vi "Analog Write N Chans.vi"(7 "Analog Ref Override":dbl, 8 "Error In":errorcluster, 9 "AO Values":dbl[](array[numeric]), 10 "AO Channel(s)":u8[](array[numeric]), 11 "LINX Resource":T1) -> (0 "Error Out":errorcluster, 3 "LINX Resource":T1)   [LabVIEW 2014, in "LMH-LINX.lvlib"]
doc: "Write value(s) to the specified analog output channel(s)."
uses:
  <vilib>/MakerHub/LINX/LMH-LINX.lvlib
  <vilib>/MakerHub/LINX/Private/Type Defs/LINX Ref.ctl
  <vilib>/MakerHub/LINX/Private/Type Defs/Platform.ctl
  <vilib>/MakerHub/LINX/Private/Type Defs/Interface.ctl
  <vilib>/MakerHub/LINX/Private/Device/Type Defs/LINX Device Config.ctl
  <vilib>/MakerHub/LINX/Private/Device/Type Defs/TCP Config.ctl
  <vilib>/MakerHub/LINX/Private/Device/Type Defs/Channels.ctl
  <vilib>/MakerHub/LINX/Private/Type Defs/Peripheral.ctl
  <vilib>/MakerHub/LINX/Private/Utilties/Generate Error.vi
  <vilib>/myRIO/Common/Instrument Driver Framework/myRIO v1.0/AO/vis/myRIO v1.0 Write AO.vi
  <vilib>/Utility/error.llb/Error Cluster From Error Code.vi
  <vilib>/MakerHub/LINX/Private/myRIO/myRIO.lvlib
  <vilib>/MakerHub/LINX/Private/Device/Device.lvlib
  <vilib>/myRIO/Instrument Drivers/Onboard IO/AO/AO.lvlib
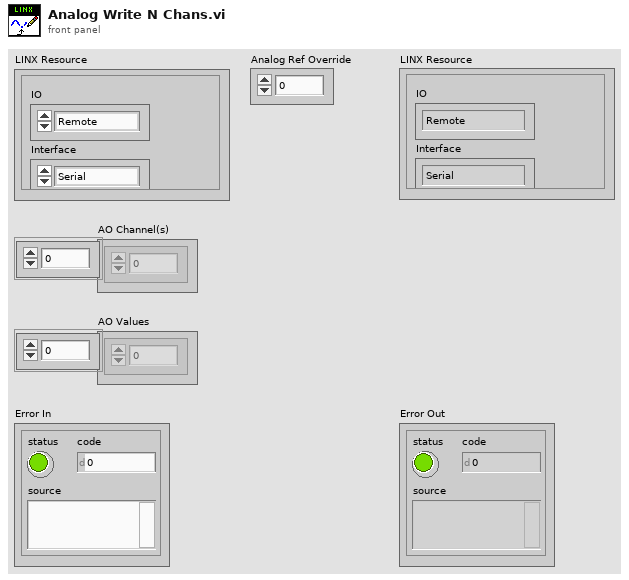
[diagram p1: front panel]
types:
  T1 = typedef "LMH-LINX.lvlib/LINX Ref.ctl" = cluster{"IO":T2, "Interface":T3, "LINX Device Config":T4}
  T2 = typedef "LMH-LINX.lvlib/Platform.ctl" = enum16{"Remote", "Local"}
  T3 = typedef "LMH-LINX.lvlib/Interface.ctl" = enum16{"Serial", "TCP"}
  T4 = typedef "LMH-LINX.lvlib/Device.lvlib/LINX Device Config.ctl" = cluster{"Interface":T3, "COM Port":refnum<visa-resource-name>, "TCP Configuration":T5, "Device Family":u8, "Device ID":u8, "Device Name":string, "TCP Ref":refnum<k5>, "Channels":T6}
  T5 = typedef "LMH-LINX.lvlib/Device.lvlib/TCP Config.ctl" = cluster{"IP Address":string, "Port":u16}
  T6 = typedef "LMH-LINX.lvlib/Channels.ctl" = cluster{"DI":u8[], "DO":u8[], "AI":u8[], "AO":u8[], "PWM":u8[], "QE":u8[], "UART":u8[], "I2C 2":u8[], "SPI":u8[], "CAN":u8[], "Servo":u8[], "AI Ref (V)":dbl, "AI Resolution (Bits)":u8, "AO Ref (V)":dbl, "AO Resolution (Bits)":u8}
  T7 = typedef "LMH-LINX.lvlib/Peripheral.ctl" = enum8{"DI", "DO", "AI", "AO", "PWM", "QE", "UART", "I2C", "SPI", "CAN", "Servo"}
  T8 = typedef "AO.lvlib/AO Reference.ctl" = cluster{"myRIO Reference":T9, "AO Channel List":T13, "AO Scaling Constant List":T15}
  T9 = typedef "myRIO Generic Hardware Reference.ctl" = cluster{"myRIO Model":T10, "myRIO Hardware Reference":T11}
  T10 = typedef "Hardware Version Enum.ctl" = enum16{"Unknown", "myRIO-1900", "myRIO-1950"}
  T11 = typedef "myRIO v1.0 Reference.ctl" = cluster{"Generic FPGA Reference":T12, "Allow multiple opens":bool}
  T12 = typedef "Generic FPGA Reference.ctl" = refnum<k20>
  T13 = typedef "AO Channels List.ctl" = T14[]
  T14 = typedef "AO Channels Enum.ctl" = enum16{"Not Connected", "AudioOut/Left", "AudioOut/Right", "C/AO0", "C/AO1", "A/AO0", "A/AO1", "B/AO0", "B/AO1"}
  T15 = typedef "Analog Scaling Constants List.ctl" = T16[]
  T16 = typedef "Analog Scaling Constants.ctl" = cluster{"LSB Weight (Volts)":dbl, "Offset (Volts)":dbl, "Signed?":bool}
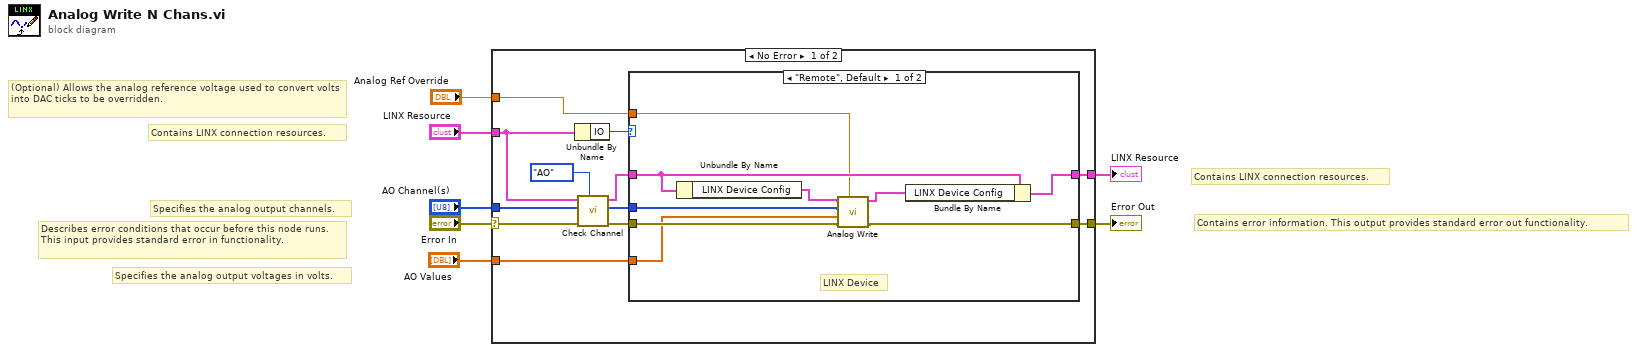
[diagram p0: block diagram]
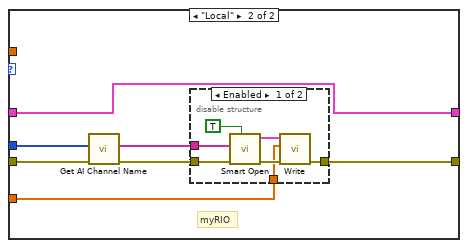
[diagram p2: hidden frame]
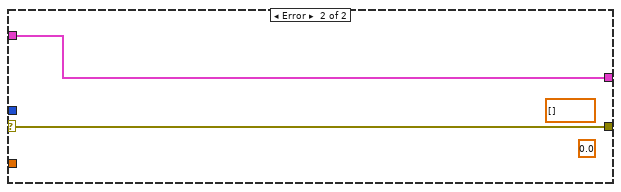
[diagram p4: hidden frame]
diagram:
  # "Contains LINX connection resources."
  # "Contains error information. This output provides standard error out functionality."
  # "Specifies the analog output voltages in volts."
  # "Specifies the analog output channels."
  # "(Optional) Allows the analog reference voltage used to convert volts into DAC ticks to be overridden."
  # "Contains LINX connection resources."
  # "Describes error conditions that occur before this node runs. This input provides standard error in functionality."
  n1 = case shown="No Error" "Error In" {
    selector: "Error In" -> [w9 w45]
    tunnel: [w18 w45] -> w7
    tunnel: [w17 w44] -> w6
    tunnel: "LINX Resource" -> [w12 w44]
    tunnel: "AO Channel(s)" -> [w11 _]
    tunnel: "Analog Ref Override" -> [w10 _]
    tunnel: "AO Values" -> [w8 _]
    frame No Error {
      n2 = Unbundle By Name(w12) -> ("IO"=w19:T2)
      n3 = call <vilib>:"Check Channel.vi"("Peripheral"=Peripheral."AO", "Error In"=w9, "Channels"=w11, "LINX Resource"=w12) -> ("Error Out"=w16:errorcluster, "Channels"=w15:u8[], "LINX Resource"=w13:T1)  [unwired: 5 in]
      n4 = case shown="\"Remote\", Default" w19 {
        tunnel: w16 -> [w23 w31]
        tunnel: w13 -> [w28 w35]
        tunnel: [w24 w33] -> w18
        tunnel: [w27 w35] -> w17
        tunnel: w15 -> [w22 w34]
        tunnel: w10 -> [w20 _]
        tunnel: w8 -> [w21 w29]
        frame "Remote", Default {
          # "LINX Device"
          n5 = Unbundle By Name(w28) -> ("LINX Device Config"=w26:T4)
          n6 = call <vilib>:"Analog Write.vi"("Analog Ref Override"=w20, "Error In"=w23, "AO Values"=w21, "AO Channels"=w22, "LINX Device Config"=w26) -> ("Error Out"=w24:errorcluster, "LINX Device Config"=w25:T4)  [unwired: 5 in]
          n7 = Bundle By Name(cluster=w28, "LINX Device Config"=w25) -> (w27:T1)
        }
        frame "Local" {
          # "myRIO"
          n8 = call <vilib>:"Get AI Channel Name.vi"("Error In"=w31, "AI Channel Nums"=w34) -> ("Error Out"=w30:errorcluster, "AI Channels"=w32:string[])  [unwired: 7 in]
          n9 = disable-structure shown="Enabled" {
            disable-tunnel: w30 -> [w39 w43]
            disable-tunnel: [w37 w43] -> w33
            disable-tunnel: w32 -> [w38 _]
            disable-tunnel: w29 -> [w36 _]
            frame Enabled {
              n10 = call <vilib>:"Smart Open.vi"("Allow multiple opens?"=TRUE, "error in (no error)"=w39, "Channel Names"=w38) -> ("error out"=w41:errorcluster, "AO Ref Out"=w42:T8)  [unwired: 7 in]
              n11 = call <vilib>:"Write.vi"("error in (no error)"=w41, "Values"=w36, "AO Ref In"=w42) -> ("error out"=w37:errorcluster)  [unwired: 6 in, 1 out]
            }
            frame Disabled {
            }
          }
        }
      }
    }
    frame Error {
      (unwired) 0.0 ("AI Ref")
      (unwired) dbl[] [] ("Values")
    }
  }
  "Error Out" <- w7
  "LINX Resource" <- w6
